vi "IP Ping Moniter.vi"(8 "error in (no error)":errorcluster, 11 "IP/Address":string="127.0.0.1") -> (0 "error out":errorcluster, 2 "Sucessful?":bool, 3 "Status":i32(ring) items=["Success"=0, "DestinationNetworkUnreachable"=11002, "DestinationHostUnreachable"=11003, "DestinationProhibited, DestinationProtocolUnreachable"=11004, "DestinationPortUnreachable"=11005, "NoResources"=11006, "BadOption"=11007, "HardwareError"=11008, "PacketTooBig"=11009, "TimedOut"=11010, "BadRoute"=11012, "TtlExpired"=11013, "TtlReassemblyTimeExceeded"=11014, "ParameterProblem"=11015, "SourceQuench"=11016, "BadDestination"=11018, "DestinationUnreachable"=11040, "TimeExceeded"=11041, "BadHeader"=11042, "UnrecognizedNextHeader"=11043, "IcmpError"=11044, "DestinationScopeMismatch"=11045, "Unknown"=-1])   [LabVIEW 2023, in "HardwareAbstractionLayer_LVOOP.lvlib" / "Wait Monitor.lvclass"]
uses:
  Wait Monitor.lvclass
panel:
  out "RoundtripTime":i64
  in  "timeout":i32=2000
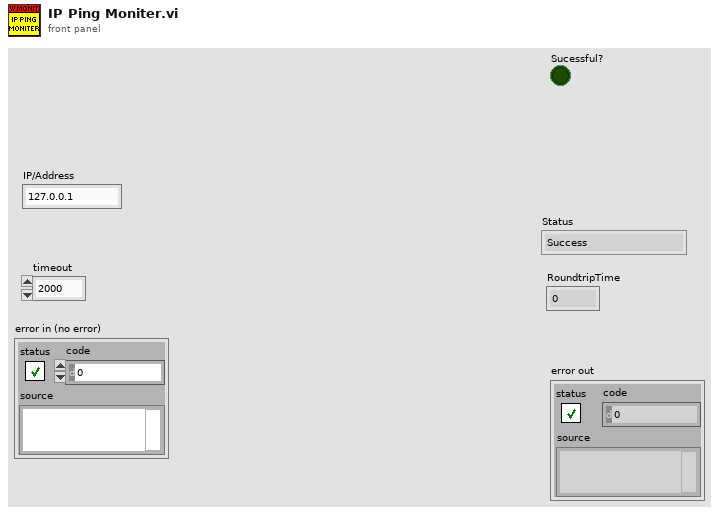
[diagram p1: front panel]
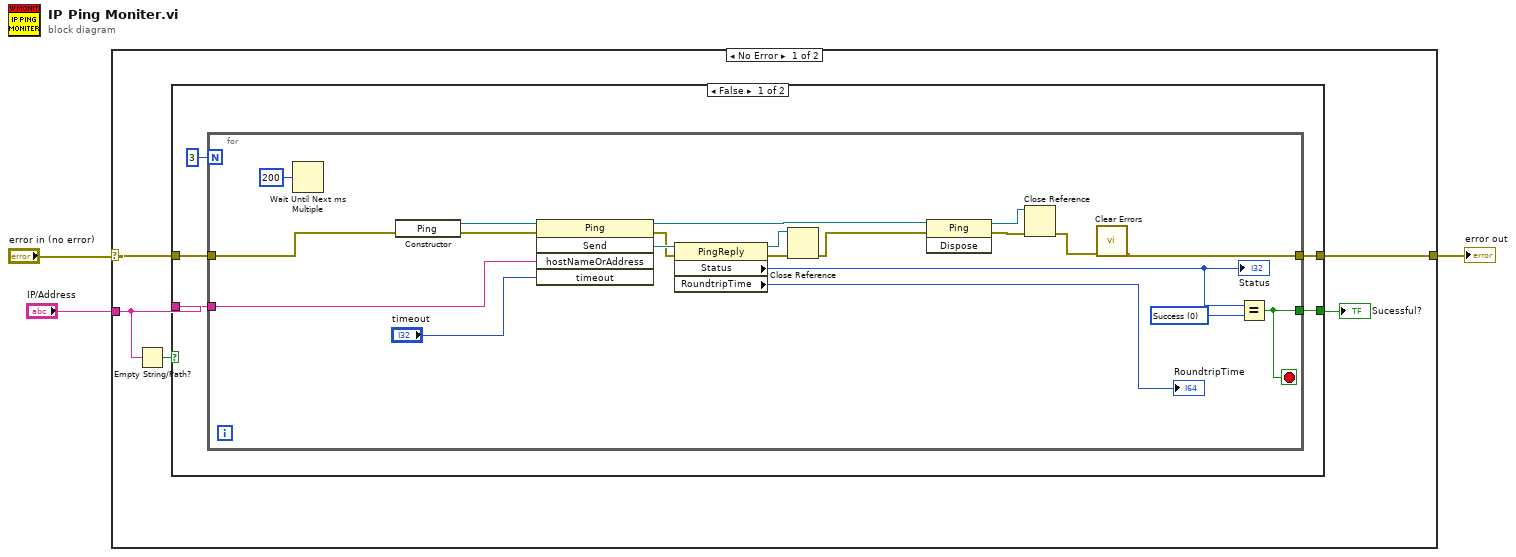
[diagram p0: block diagram]
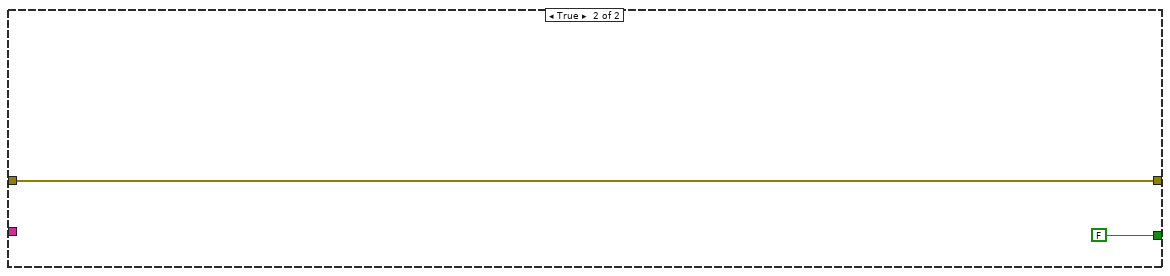
[diagram p2: hidden frame]
diagram:
  n1 = case shown="No Error" "error in (no error)" {
    selector: "error in (no error)" -> [w6 w36]
    tunnel: "IP/Address" -> [w5 _]
    tunnel: [w7 w36] -> w2
    frame No Error {
      n2 = Empty String/Path?(string/path=w5) -> (empty?=w4:bool)
      n3 = case shown="False" w4 {
        tunnel: [w13 FALSE] -> w8
        tunnel: [w12 w35] -> w7
        tunnel: w6 -> [w11 w35]
        tunnel: w5 -> [w10 _]
        frame False {
          n4 = for {
            N: 3 -> [_]
            tunnel: [w18] -> w13
            tunnel: w10 -> [w17]
            tunnel: w11 -> [w15]
            tunnel: [w14] -> w12
            stop <- w18 stop-if-true
            w20 = 0 items=["Success"=0, "DestinationNetworkUnreachable"=11002, "DestinationHostUnreachable"=11003, "DestinationProhibited, DestinationProtocolUnreachable"=11004, "DestinationPortUnreachable"=11005, "NoResources"=11006, "BadOption"=11007, "HardwareError"=11008, "PacketTooBig"=11009, "TimedOut"=11010, "BadRoute"=11012, "TtlExpired"=11013, "TtlReassemblyTimeExceeded"=11014, "ParameterProblem"=11015, "SourceQuench"=11016, "BadDestination"=11018, "DestinationUnreachable"=11040, "TimeExceeded"=11041, "BadHeader"=11042, "UnrecognizedNextHeader"=11043, "IcmpError"=11044, "DestinationScopeMismatch"=11045, "Unknown"=-1] ("Status 2")
            n5 = Wait Until Next ms Multiple(millisecond multiple=u32 200 ("milliseconds to wait")) -> ()  [unwired: 1 out]
            n6 = constructor class="Ping"(error in=w15) -> (reference out=w29:refnum<k24>, error out=w28:errorcluster)  [unwired: 2 in, 1 out]
            n7 = invoke class="Ping" method="Send"(reference=w29, error in=w28, "hostNameOrAddress"=w17, "timeout"="timeout") -> (reference out=w27:refnum<k24>, error out=w30:errorcluster, "Send"=w31:refnum<k24>)  [unwired: 1 in, 2 out]
            n8 = property class="PingReply"(reference=w31, error in=w30) -> (reference out=w26:refnum<k24>, error out=w25:errorcluster, "Status"=w21:i32, "RoundtripTime"=→"RoundtripTime":i64)
            "Status" <- w21
            n9 = Close Reference(reference=w26, error in (no error)=w25) -> (error out=w16:errorcluster)
            n10 = invoke class="Ping" method="Dispose"(reference=w27, error in=w16) -> (reference out=w23:refnum<k24>, error out=w24:errorcluster)  [unwired: 1 in, 1 out]
            n11 = Close Reference(reference=w23, error in (no error)=w24) -> (error out=w22:errorcluster)
            n12 = call <vilib>:"Clear Errors.vi"("error in (no error)"=w22) -> ("error out"=w14:errorcluster)  [unwired: 5 in, 1 out]
            n13 = Equal?(x=w21, y=w20) -> (x = y?=w18:bool)
          }
        }
        frame True {
        }
      }
      "Sucessful?" <- w8
    }
    frame Error {
    }
  }
  "error out" <- w2
